vi "topicRequest.vi"(1 "XML":string) -> (0 "Subscriber":T1)   [LabVIEW 2018]
doc: "Takes XML from a topic request and returns a cluster with \n-Caller ID\n-Topic name\n-Protocol\n-URI\n-TCP ID"
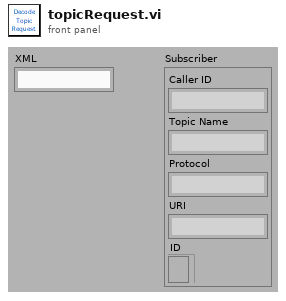
[diagram p1: front panel]
types:
  T1 = cluster{"Caller ID":string, "Topic Name":string, "Protocol":string, "URI":string, "ID":refnum<k5>}
  T2 = cluster{"Caller ID":string, "Topic Name":string, "Protocol":string, "Caller ID 2":string, "ID":refnum<k5>}
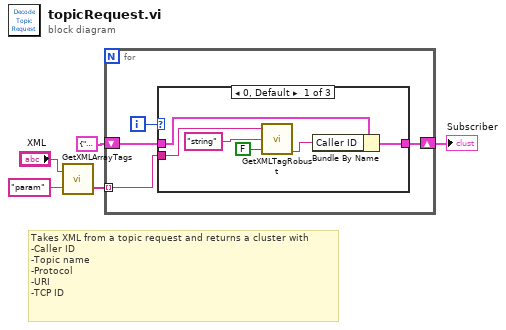
[diagram p0: block diagram]
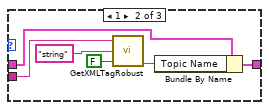
[diagram p2: hidden frame]
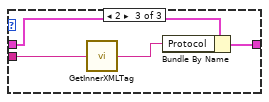
[diagram p3: hidden frame]
diagram:
  # "Takes XML from a topic request and returns a cluster with \n-Caller ID\n-Topic name\n-Protocol\n-URI\n-TCP ID"
  n1 = call <userlib>:"GetXMLArrayTags.vi"("ArrayTag"="param", "String"="XML") -> ("Array"=w3:string[])  [unwired: 1 out]
  n2 = for {
    tunnel: w3 -> [w7] mode=indexing
    shift-right: [w6] -> w5
    shift-left: T2 {"Caller ID"="", "Topic Name"="", "Protocol"="", "Caller ID 2"="", "ID"=refnum} ("Subscriber") -> [w8]
    i -> [w9]
    n3 = case shown="0, Default" w9 {
      tunnel: w8 -> [w13 w21 w23]
      tunnel: w7 -> [w15 w19 w25]
      tunnel: [w11 w20 w22] -> w6
      frame 0, Default {
        n4 = call <userlib>:"GetXMLTagRobust.vi"("Tag only? (T)"=FALSE ("Tag only?"), "Tag"="string", "String"=w15) -> ("value"=w12:string)  [unwired: 3 out]
        n5 = Bundle By Name(cluster=w13, "Caller ID"=w12) -> (w11:T2)
      }
      frame 1 {
        n6 = call <userlib>:"GetXMLTagRobust.vi"("Tag only? (T)"=FALSE ("Tag only?"), "Tag"="string", "String"=w19) -> ("value"=w16:string)  [unwired: 3 out]
        n7 = Bundle By Name(cluster=w21, "Topic Name"=w16) -> (w20:T2)
      }
      frame 2 {
        n8 = call <userlib>:"GetInnerXMLTag.vi"("String"=w25) -> ("Value"=w24:string)
        n9 = Bundle By Name(cluster=w23, "Protocol"=w24) -> (w22:T2)
      }
    }
  }
  "Subscriber" <- w5
